vi "getLocalRepoId.vi"(8 "error in (no error)":errorcluster, 11 "hgHandler in":refnum<class "hgHandler.lvclass">) -> (0 "error out":errorcluster, 1 "Log":string, 3 "hgHandler out":refnum<class "hgHandler.lvclass">, 4 "ID":string)   [LabVIEW 2013, in "hgHandler.lvclass"]
uses:
  hgHandler.lvclass
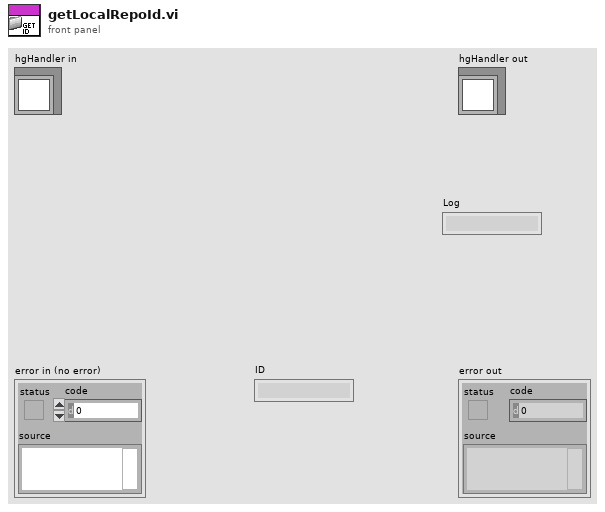
[diagram p1: front panel]
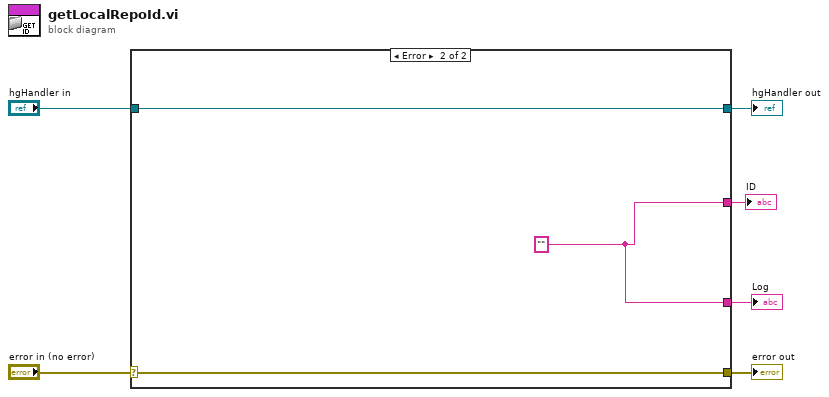
[diagram p0: block diagram]
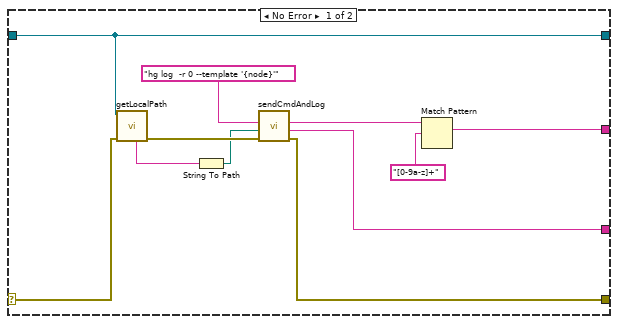
[diagram p2: hidden frame]
diagram:
  n1 = case shown="Error" "error in (no error)" {
    selector: "error in (no error)" -> [w12 w20]
    tunnel: [w15 w20] -> w5
    tunnel: [w13 w19] -> w3
    tunnel: "hgHandler in" -> [w13 w19]
    tunnel: [w16 w18] -> w2
    tunnel: [w7 w18] -> w1
    frame No Error {
      n2 = call-dynamic "getLocalPath.vi"("error in (no error)"=w12, "repoHandler in"=w13) -> ("error out"=w11:errorcluster, "Local Path"=w10:string)  [unwired: 7 in, 1 out]
      n3 = String To Path(string=w10) -> (path=w9:path)
      n4 = call "sendCmdAndLog.vi"("error in (no error)"=w11, "working directory"=w9, "command"="hg log  -r 0 --template '{node}'" ("command line")) -> ("error out"=w15:errorcluster, "Log"=w7:string, "standard output"=w14:string)  [unwired: 6 in]
      n5 = Match Pattern(string=w14, regular expression="[0-9a-z]+") -> (match substring=w16:string)  [unwired: 1 in, 3 out]
    }
    frame Error {
      w18 = "" ("standard output")
    }
  }
  "error out" <- w5
  "hgHandler out" <- w3
  "Log" <- w1
  "ID" <- w2
